vi "Write Display - Description.vi"(8 "error in (no error)":errorcluster, 10 "description":string, 11 "NT Base in":refnum<class "NT Base.lvclass">) -> (0 "error out":errorcluster, 3 "NT Base out":refnum<class "NT Base.lvclass">)   [LabVIEW 2020, in "PV Access.lvlib" / "PV Data.lvlib" / "NT Base.lvclass"]
uses:
  NT Base.lvclass
  NT Base.lvclass/NT Base.ctl
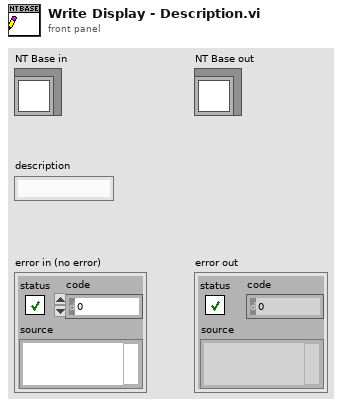
[diagram p1: front panel]
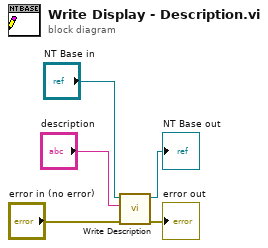
[diagram p0: block diagram]
diagram:
  n1 = call-dynamic "Write Description.vi"("error in (no error)"="error in (no error)", "description"="description", "Base Interface in"="NT Base in") -> ("error out"=→"error out":errorcluster, "Base Interface out"=→"NT Base out":refnum<class "NT Base.lvclass">)  [unwired: 7 in]
